vi "Initialize.vi"(7 "UI Interaction":refnum<class "UI Interaction.lvclass">, 8 "error in (no error)":errorcluster {"code" format="Error %.0f"}, 10 "Settings Path":path, 11 "VIDoc Printer In":refnum<class "VIDoc Printer.lvclass">) -> (0 "error out":errorcluster {"code" format="Error %.0f"}, 3 "VIDoc Printer Out":refnum<class "VIDoc Printer.lvclass">)   [LabVIEW 2023, in "VIDoc Printer.lvlib" / "VIDoc Printer.lvclass"]
doc: "Initialize Printer, load in Printer specific settings, start connections, etc."
uses:
  VIDoc Printer.lvclass
  <vilib>/DMC/VIDoc/Framework/UI Interaction/Interface/UI Interaction.lvclass
  VIDoc Printer.lvclass/VIDoc Printer.ctl
  Settings/Printer Settings/Printer Settings.lvclass
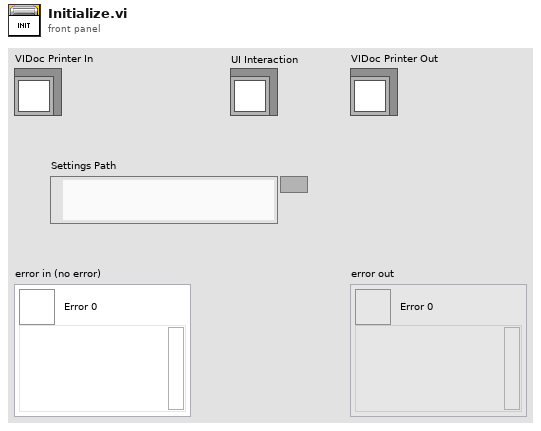
[diagram p1: front panel]
types:
  T1 = typedef "VIDoc Printer.lvlib/Printer Settings.lvclass/Printer Settings Cluster.ctl" = cluster{"Project":T2, "VI Member":T3, "Interface":T5, "Class":T7, "Library":T8, "Control Member":T9, "Format Options":T10, "Library Scope":cluster{"Public":bool, "Community":bool, "Private":bool, "Unknown":bool}, "LLB":T13, "Bookmark Settings Map":map{string, T3}}
  T2 = typedef "VIDoc Printer.lvlib/Printer Settings.lvclass/Project Settings.ctl" = cluster{"Paths":bool, "Descriptions":bool, "Memory":bool, "Options":bool, "Symbols":bool}
  T3 = typedef "VIDoc Printer.lvlib/Printer Settings.lvclass/VI Settings.ctl" = cluster{"Memory":bool, "By Folder":bool, "By Tree":bool, "By List":bool, "Methods":bool, "Method Options":cluster{"Front Panels":bool, "Options":bool, "Controls":bool}, "List Detail Level":T4, "Methods Detail Level":T4, "Controls Detail Level":T4}
  T4 = typedef "VIDoc Printer.lvlib/Printer Settings.lvclass/Detail Level Enum.ctl" = enum16{"None", "Minimal", "Standard", "Full"}
  T5 = typedef "VIDoc Printer.lvlib/Printer Settings.lvclass/Interface Settings.ctl" = cluster{"Memory":bool, "By List":bool, "Details":bool, "Detail Options":cluster{"Description":bool, "Properties":bool, "Inheritance":bool, "Inheritance Options":cluster{"Parent Interfaces":bool, "Friends":bool}}, "List Detail Level":T4, "Controls Detail Level":T4, "Methods Detail Level":T4, "Controls Scope":T6, "Methods Scope":T6}
  T6 = typedef "VIDoc Printer.lvlib/Printer Settings.lvclass/Scope Settings.ctl" = cluster{"Public":bool, "Protected":bool, "Community":bool, "Private":bool, "Unknown":bool}
  T7 = typedef "VIDoc Printer.lvlib/Printer Settings.lvclass/Class Settings.ctl" = cluster{"Memory":bool, "By Folder":bool, "By Tree":bool, "By List":bool, "Details":bool, "Detail Options":cluster{"Description":bool, "Properties":bool, "Inheritance":bool, "Inheritance Options":cluster{"Parent Classes":bool, "Parent Interfaces":bool, "Parent Libraries":bool, "Friends":bool}}, "CPD Detail Level":T4, "List Detail Level":T4, "Controls Detail Level":T4, "Methods Detail Level":T4, "Set Accessor Detail Level":T4, "Get Accessor Detail Level":T4, "Controls Scope":T6, "Methods Scope":T6, "Get Accessors Scope":T6, "Set Accessors Scope":T6}
  T8 = typedef "VIDoc Printer.lvlib/Printer Settings.lvclass/Library Settings.ctl" = cluster{"Memory":bool, "By Folder":bool, "By Tree":bool, "By List":bool, "Details":bool, "Detail Options":cluster{"Description":bool, "Properties":bool, "Friends":bool, "Child Libraries":bool}, "List Detail Level":T4, "Methods Detail Level":T4, "Controls Detail Level":T4, "Methods Scope":T6, "Controls Scope":T6}
  T9 = typedef "VIDoc Printer.lvlib/Printer Settings.lvclass/Control Settings.ctl" = cluster{"Memory":bool, "By Folder":bool, "By Tree":bool, "By List":bool, "Controls":bool, "List Detail Level":T4, "Controls Detail Level":T4}
  T10 = typedef "VIDoc Printer.lvlib/Printer Settings.lvclass/Formatting Options.ctl" = cluster{"Background":cluster{"Public Scope":T11, "Protected Scope":T11, "Community Scope":T11, "Private Scope":T11, "Unknown Scope":T11, "Auto Error Handling":T11, "Inline":T11, "Separate CC":T11, "Execution Priority Normal":T11, "Reentrancy Non-RE":T11}, "Bookmark Options":T12}
  T11 = typedef "VIDoc Printer.lvlib/Printer Settings.lvclass/Background Formatting Cluster.ctl" = cluster{"Option":bool, "Color":u32, "Operator":bool}
  T12 = typedef "VIDoc Printer.lvlib/Printer Settings.lvclass/Bookmark Options.ctl" = cluster{"Bookmarks as New Line in VI Descriptions":bool, "Unique Bookmark Tags Only":bool, "Include Tag and Text":bool}
  T13 = typedef "VIDoc Printer.lvlib/Printer Settings.lvclass/LLB Settings.ctl" = cluster{"Methods":bool, "Controls":bool, "Methods Detail Level":T4, "Controls Detail Level":T4}
  T14 = typedef "VIDoc Printer.lvlib/Printer Settings.lvclass/Enabled Sections Cluster.ctl" = cluster{"Projects":bool, "Interfaces":bool, "Classes":bool, "Libraries":bool, "VIs":bool, "Controls":bool, "LLBs":bool}
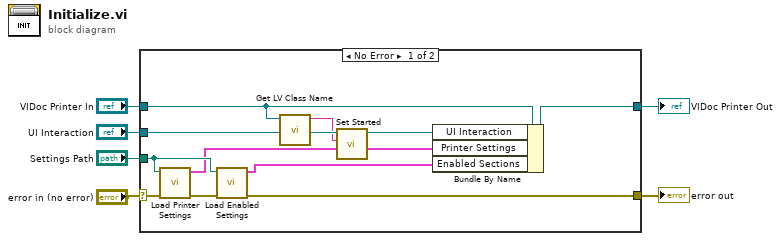
[diagram p0: block diagram]
diagram:
  n1 = case shown="No Error" "error in (no error)" {
    selector: "error in (no error)" -> [w16 w19]
    tunnel: [w7 w19] -> w5
    tunnel: [w17 w18] -> w3
    tunnel: "VIDoc Printer In" -> [w9 w18]
    tunnel: "UI Interaction" -> [w11 _]
    tunnel: "Settings Path" -> [w14 _]
    frame No Error {
      n2 = call "Load Printer Settings.vi"("Error in"=w16, "Settings Path"=w14) -> ("Error out"=w15:errorcluster, "Printer Settings"=w13:T1)  [unwired: 7 in, 1 out]
      n3 = call "Load Enabled Settings.vi"("Error in"=w15, "Settings Path"=w14) -> ("Error out"=w7:errorcluster, "Enabled Sections"=w12:T14)  [unwired: 7 in, 1 out]
      n4 = call <vilib>:"Get LV Class Name.vi"("object"=w9) -> ("class name"=w8:string)  [unwired: 9 in, 1 out]
      n5 = call-dynamic "Set Started.vi"("Process"=w8, "UI Interaction in"=w11) -> ("UI Interaction out"=w10:refnum<class "UI Interaction.lvclass">)  [unwired: 8 in, 1 out]
      n6 = Bundle By Name(cluster=w9, "UI Interaction"=w10, "Printer Settings"=w13, "Enabled Sections"=w12) -> (w17:refnum<class "VIDoc Printer.lvclass">)
    }
    frame Error {
    }
  }
  "error out" <- w5
  "VIDoc Printer Out" <- w3
